vi "GetClassName.vi"(0 "reference in":refnum<class "G#Interface.lvclass">, 5 "error in (no error)":errorcluster) -> (14 "reference out":refnum<class "G#Interface.lvclass">, 15 "class name":string, 16 "lvlib hierarchy":string[](array[string]), 17 "full class name":string, 19 "error out":errorcluster)   [LabVIEW 2020, in "G#Interface.lvclass"]
doc: "Returns the class name, full class name , lvlib hierarchy for the specified object."
uses:
  G#Interface.lvclass
  G#Interface.lvclass/G#Interface.ctl
  G#Object/G#Object.lvclass
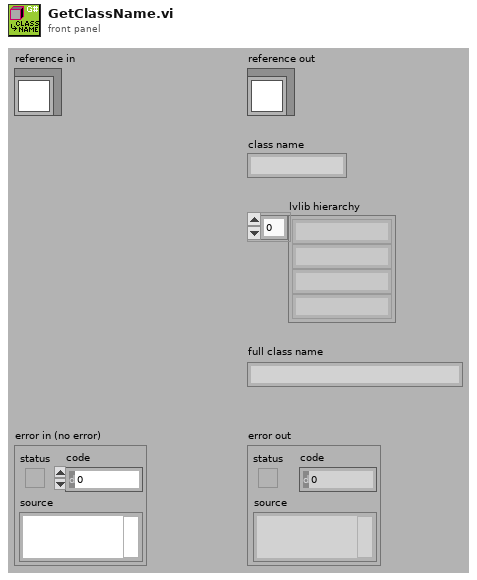
[diagram p1: front panel]
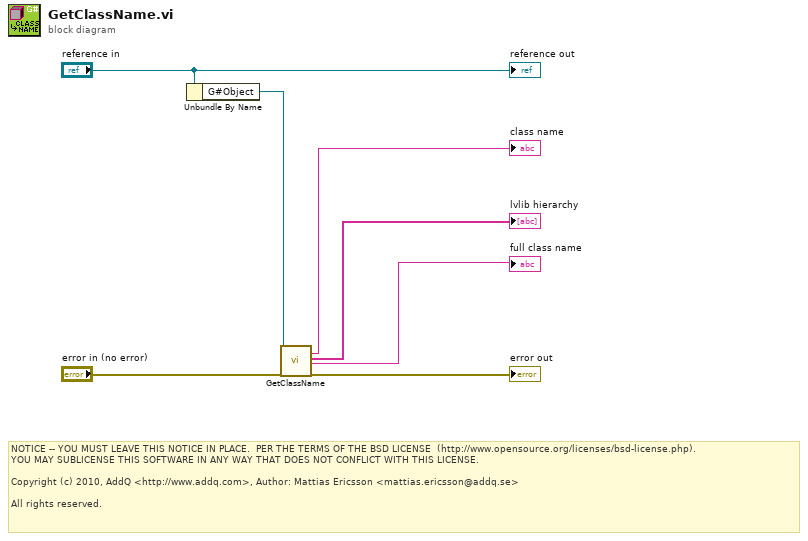
[diagram p0: block diagram]
diagram:
  # "NOTICE -- YOU MUST LEAVE THIS NOTICE IN PLACE.  PER THE TERMS OF THE BSD LICENSE  (http://www.opensource.org/licenses/bsd-license.php).\nYOU MAY SUBLICENSE THIS SOFTWARE IN ANY WAY THAT DOES NOT CONFLICT WITH THIS LICENSE.\n\nCopyright (c) 2010, AddQ <http://www.addq.com>, Author: Mattias Ericsson <mattias.ericsson@addq.se>\n\nAll rights reserved."
  n1 = Unbundle By Name("reference in") -> ("G#Object"=w5:refnum<class "G#Object.lvclass">)
  n2 = call-dynamic "GetClassName.vi"("reference in"=w5, "error in (no error)"="error in (no error)") -> ("class name"=→"class name":string, "lvlib hierarchy"=→"lvlib hierarchy":string[], "full class name"=→"full class name":string, "error out"=→"error out":errorcluster)  [unwired: 13 in, 1 out]
  "reference out" <- "reference in"
